vi "Close.vi"(8 "error in (no error)":errorcluster, 11 "TestExec in":refnum<class "TestExec.lvclass">) -> (0 "error out":errorcluster, 3 "TestExec out":refnum<class "TestExec.lvclass">)   [LabVIEW 2021, in "TestExec.lvclass"]
uses:
  TestExec.lvclass
  TestExec.lvclass/TestExec.ctl
  <vilib>/addons/TestStand/_TSUtility.llb/TestStand - Set Property Value (Boolean).vi
  OPC UA/OPC UA.lvclass
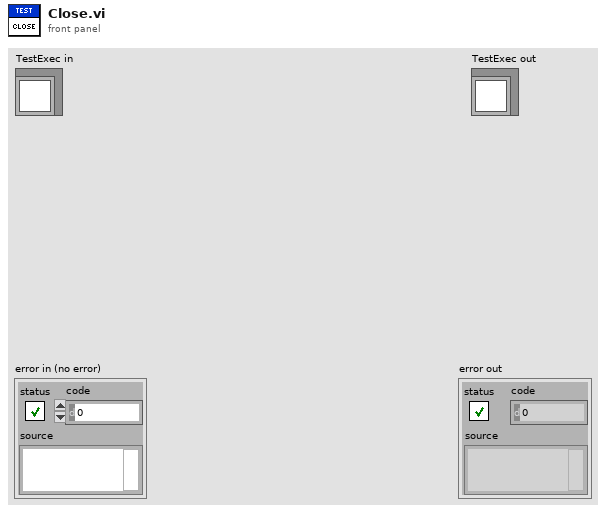
[diagram p1: front panel]
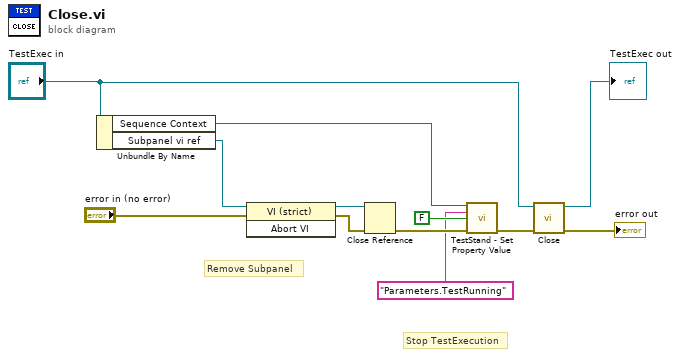
[diagram p0: block diagram]
diagram:
  # "Stop TestExecution"
  # "Remove Subpanel"
  n1 = Unbundle By Name("TestExec in") -> ("Sequence Context"=w4:refnum<k7>, "Subpanel vi ref"=w2:refnum<vi>)
  n2 = invoke on="Invoke Node" class="VI (strict)" method="Abort VI"(reference=w2, error in="error in (no error)") -> (reference out=w5:refnum<vi>, error out=w7:errorcluster)  [unwired: 1 in, 1 out]
  n3 = Close Reference(reference=w5, error in (no error)=w7) -> (error out=w10:errorcluster)
  n4 = call-poly <vilib>:"TestStand - Set Property Value.vi"("Sequence Context In"=w4, "Lookup String"="Parameters.TestRunning", "New Value"=FALSE ("Insert If Missing"), "error in (no error)"=w10) -> ("error out"=w3:errorcluster)  [unwired: 10 in, 1 out]
  n5 = call-parent "Close.vi"("error in (no error)"=w3, "OPC UA in"="TestExec in") -> ("error out"=→"error out":errorcluster, "OPC UA out"=→"TestExec out":refnum<class "TestExec.lvclass">)  [unwired: 8 in]
